vi "while_tunel.vi"() -> ()   [LabVIEW 2020]
panel:
  in  "stop":bool
  out "Numeric 3":dbl
  in  "Numeric 2":dbl
  in  "Numeric":dbl
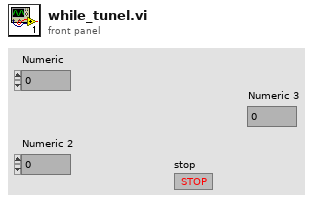
[diagram p1: front panel]
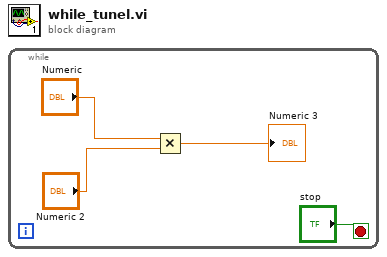
[diagram p0: block diagram]
diagram:
  n1 = while {
    stop <- "stop" stop-if-true
    n2 = Multiply(x="Numeric", y="Numeric 2") -> (x*y=→"Numeric 3":dbl)
  }
